vi "FTDI_Parse_Error_Code.vi"(8 "error in (no error)":errorcluster, 11 "FT_Status":u32) -> (0 "error out":errorcluster)   [LabVIEW 2016]
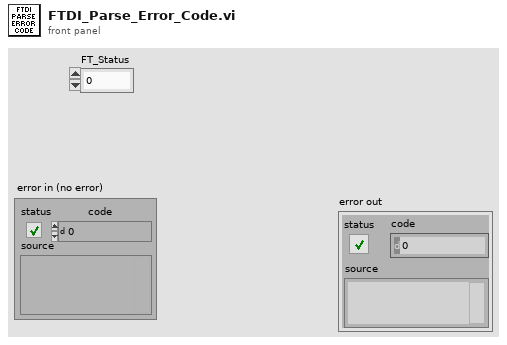
[diagram p1: front panel]
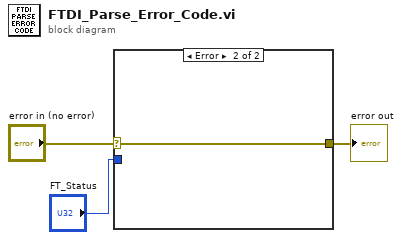
[diagram p0: block diagram]
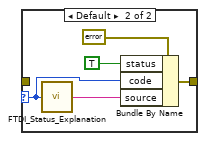
[diagram p3: hidden frame]
diagram:
  n1 = case shown="Error" "error in (no error)" {
    selector: "error in (no error)" -> [w4 w13]
    tunnel: "FT_Status" -> [w6 _]
    tunnel: [w5 w13] -> w1
    frame No Error {
      n2 = case shown="0" w6 {
        selector: w6 -> [_ w11]
        tunnel: [w7 w9] -> w5
        tunnel: w4 -> [w7 _]
        frame 0 {
        }
        frame Default {
          n3 = call "FTDI_Status_Explanation.vi"("FT_Status"=w11) -> ("Status String"=w10:string)
          n4 = Bundle By Name(cluster=errorcluster {"status"=FALSE, "code"=0, "source"=""} ("error constant"), "status"=TRUE, "code"=w11, "source"=w10) -> (w9:errorcluster)
        }
      }
    }
    frame Error {
    }
  }
  "error out" <- w1
